vi "Test Criteria, Format Entry Point Table.vi"(8 "error in":errorcluster, 11 "Tbl Refnum":refnum<vi>) -> (0 "error out":errorcluster, 3 "Tbl Refnum out":refnum<vi>)   [LabVIEW 2010]
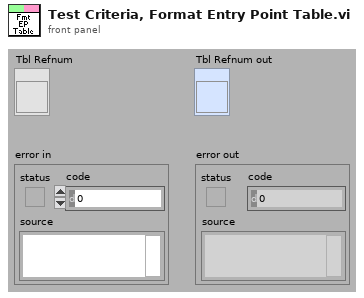
[diagram p1: front panel]
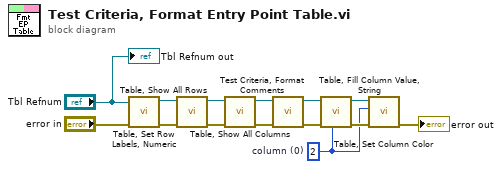
[diagram p0: block diagram]
diagram:
  w1 = 2  # column (0)
  n1 = call "Table, Set Row Labels, Numeric.vi"("error in"="error in", "Tbl Refnum"="Tbl Refnum") -> ("error out"=w13:errorcluster, "Tbl Refnum out"=w9:refnum<vi>)  [unwired: 8 in]
  n2 = call "Table, Show All Rows.vi"("error in"=w13, "Tbl Refnum"=w9) -> ("error out"=w12:errorcluster, "Tbl Refnum out"=w8:refnum<vi>)  [unwired: 8 in]
  n3 = call "Table, Show All Columns.vi"("error in"=w12, "Tbl Refnum"=w8) -> ("error out"=w10:errorcluster, "Tbl Refnum out"=w7:refnum<vi>)  [unwired: 8 in]
  n4 = call "Test Criteria, Format Comments.vi"("error in"=w10, "Tbl Refnum"=w7) -> ("error out"=w6:errorcluster, "Tbl Refnum out"=w5:refnum<vi>)  [unwired: 8 in]
  n5 = call "Table, Fill Column Value, String.vi"("column (0)"=w1, "error in"=w6, "Tbl Refnum"=w5) -> ("error out"=w4:errorcluster, "Tbl Refnum out"=w2:refnum<vi>)  [unwired: 7 in]
  n6 = call "Table, Set Column Color.vi"("error in"=w4, "col (0)"=w1, "Tbl Refnum"=w2) -> ("error out"=→"error out":errorcluster)  [unwired: 6 in, 1 out]
  "Tbl Refnum out" <- "Tbl Refnum"
